vi "VISA_smu-buffer-new_with initialization.vi"(0 "VISA resource name in":refnum<visa-resource-name>, 3 "Voltage Source Level (V)":dbl, 7 "error in (no error)":errorcluster, 12 "End voltage":ext, 14 "Initial voltage":ext, 18 "Dark Current":bool) -> (20 "VISA resource name out":refnum<visa-resource-name>, 22 "F_I_Output (A)":dbl, 23 "S_I_Output (A)":string, 24 "F_V_Output (V)":dbl, 25 "S_V_Output (V)":string, 27 "error out":errorcluster)   [LabVIEW 2014]
panel:
  out "Numeric 2":i32
  out "Exp value":ext
  out "Exp value 2":ext
  out "floor(x): largest int <= x":ext
  out "Numeric":ext
  out "abs(x)":ext
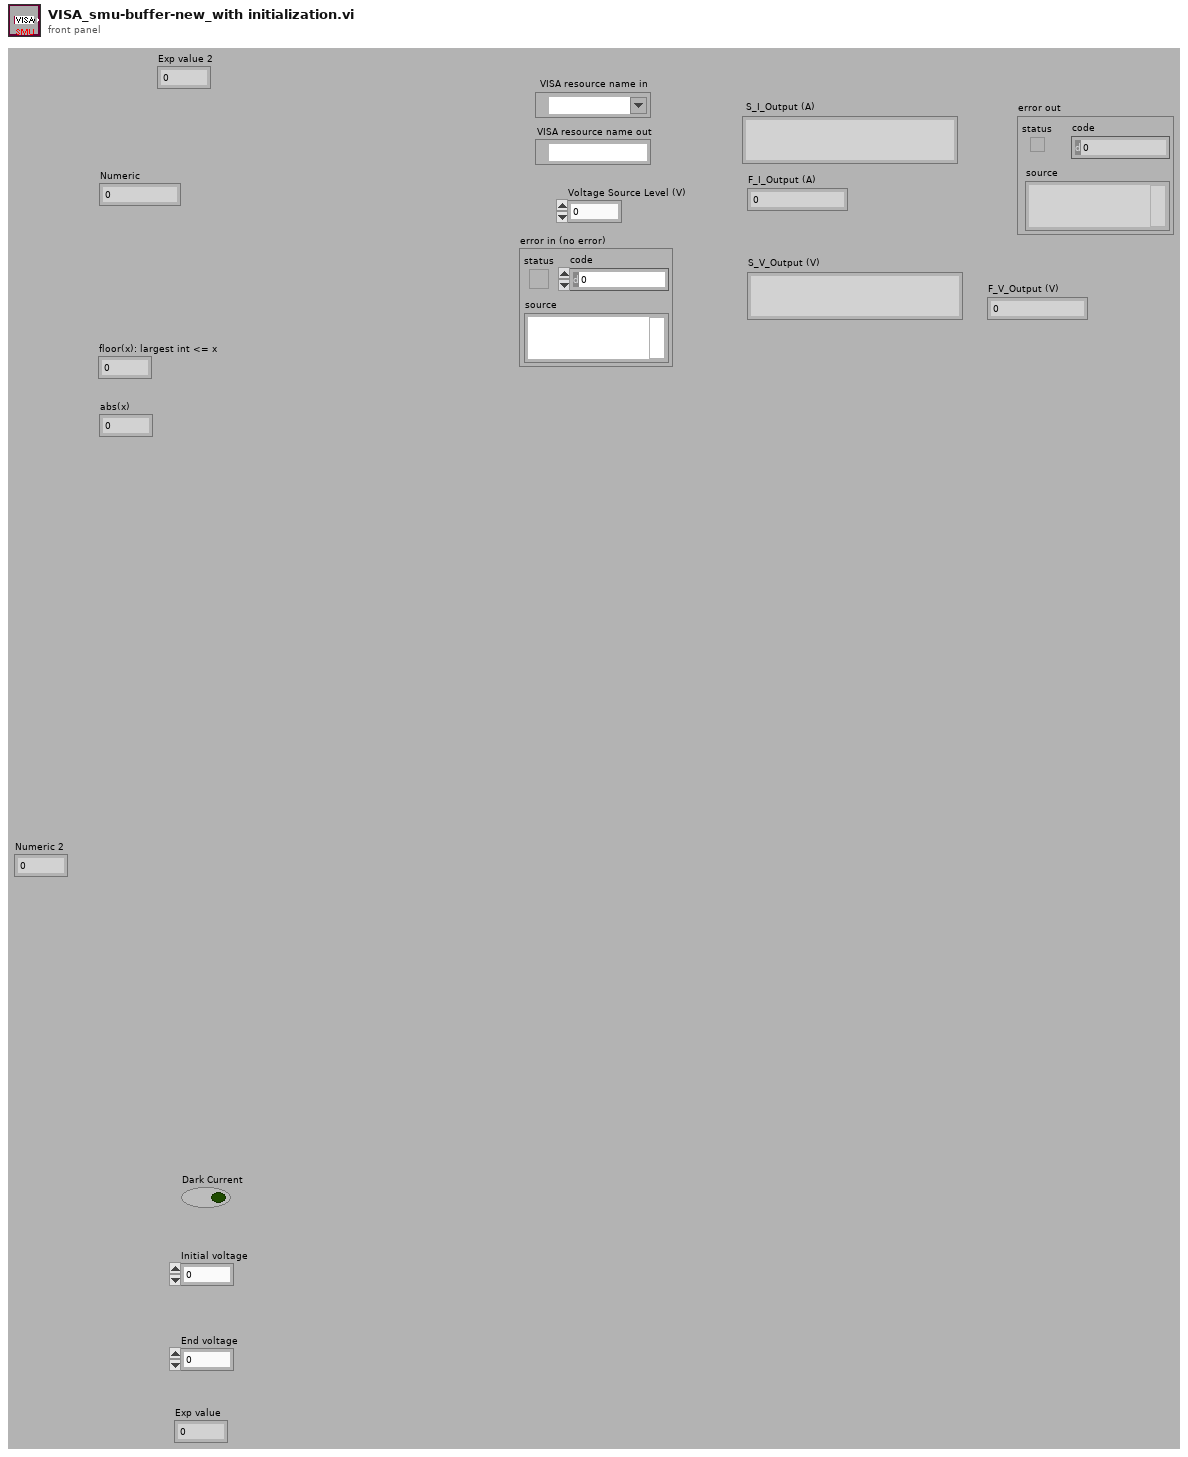
[diagram p1: front panel]
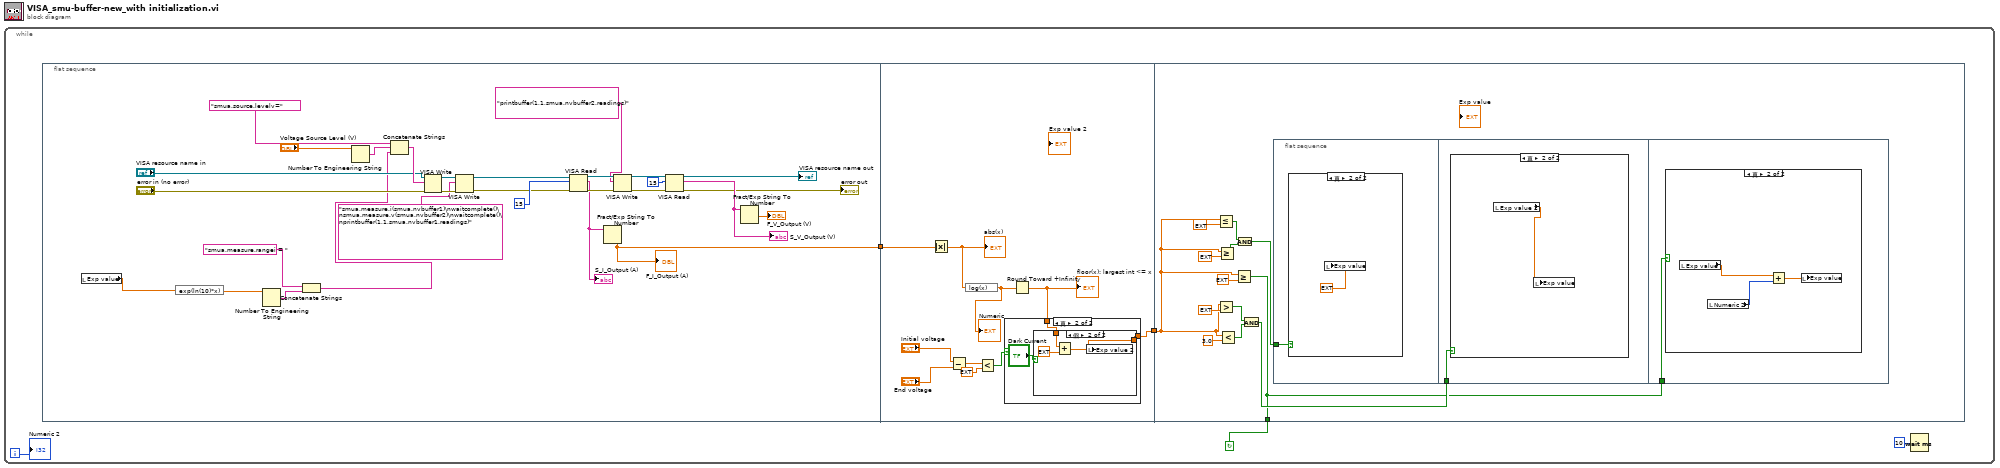
[diagram p0: block diagram]
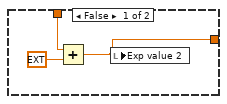
[diagram p2: hidden frame]
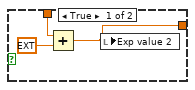
[diagram p3: hidden frame]
diagram:
  n1 = while {
    i -> [w3]
    stop <- w4 continue-if-true
    n2 = flat-sequence {
      tunnel: [w8] -> w1
      tunnel: [w40] -> w5
      tunnel: w1 -> [w41]
      tunnel: w5 -> [w58]
      tunnel: [w57] -> w4
      frame #0 {
        n3 = local read "Exp value"() -> (w6:ext)
        n4 = expression code="exp(ln(10)*x)"(w6) -> (w7:ext)
        n5 = Number To Engineering String(4:w7) -> (0:w17:string)  [unwired: 3 out]
        n6 = Concatenate Strings("smua.measure.rangei = " ("string"), w17) -> (w15:string)
        n7 = Number To Engineering String(4:"Voltage Source Level (V)") -> (0:w33:string)  [unwired: 3 out]
        n8 = Concatenate Strings("smua.source.levelv=", w33, w15) -> (w22:string)
        n9 = VISA Write(VISA resource name="VISA resource name in", write buffer=w22, error in (no error)="error in (no error)") -> (VISA resource name out=w24:refnum<visa-resource-name>, error out=w23:errorcluster)  [unwired: 1 out]
        n10 = VISA Write(VISA resource name=w24, write buffer="smua.measure.i(smua.nvbuffer1)\nwaitcomplete()\nsmua.measure.v(smua.nvbuffer2)\nwaitcomplete()\nprintbuffer(1,1,smua.nvbuffer1.readings)", error in (no error)=w23) -> (VISA resource name out=w14:refnum<visa-resource-name>, error out=w13:errorcluster)  [unwired: 1 out]
        n11 = VISA Read(VISA resource name=w14, byte count=u32 15, error in (no error)=w13) -> (VISA resource name out=w26:refnum<visa-resource-name>, read buffer=w25:string, error out=w27:errorcluster)  [unwired: 1 out]
        "S_I_Output (A)" <- w25
        n12 = Fract/Exp String To Number(string=w25) -> (number=w8:dbl)  [unwired: 4 out]
        "F_I_Output (A)" <- w8
        n13 = VISA Write(VISA resource name=w26, write buffer="printbuffer(1,1,smua.nvbuffer2.readings)", error in (no error)=w27) -> (VISA resource name out=w12:refnum<visa-resource-name>, error out=w11:errorcluster)  [unwired: 1 out]
        n14 = VISA Read(VISA resource name=w12, byte count=u32 15, error in (no error)=w11) -> (VISA resource name out=→"VISA resource name out":refnum<visa-resource-name>, read buffer=w29:string, error out=→"error out":errorcluster)  [unwired: 1 out]
        "S_V_Output (V)" <- w29
        n15 = Fract/Exp String To Number(string=w29) -> (number=→"F_V_Output (V)":dbl)  [unwired: 4 out]
      }
      frame #1 {
        n16 = Absolute Value(x=w41) -> (abs(x)=w43:dbl)
        "abs(x)" <- w43
        n17 = Subtract(x="Initial voltage", y="End voltage") -> (x-y=w37:ext)
        n18 = expression code="log(x)"(w43) -> (w44:dbl)
        "Numeric" <- w44
        n19 = Less?(x=w37, y=ext 0.0) -> (x < y?=w35:bool)
        n20 = Round Toward +Infinity(x=w44) -> (ceil(x): smallest int >= x=w42:dbl)
        "floor(x): largest int <= x" <- w42
        n21 = case shown="真" w35 {
          tunnel: w42 -> [w46 w50]
          tunnel: [w45 w49] -> w40
          frame False {
            n22 = Add(x=w46, y=ext 0.0) -> (x+y=w45:ext)
            n23 = local write "Exp value 2"(w45) -> ()
          }
          frame True {
            n24 = case shown="假" "Dark Current" {
              tunnel: w50 -> [w52 w55]
              tunnel: [w51 w54] -> w49
              frame True {
                n25 = Add(x=w52, y=ext 0.0) -> (x+y=w51:ext)
                n26 = local write "Exp value 2"(w51) -> ()
              }
              frame False {
                n27 = Add(x=w55, y=ext 1.0) -> (x+y=w54:ext)
                n28 = local write "Exp value 2"(w54) -> ()
              }
            }
          }
        }
      }
      frame #2 {
        n29 = Less Or Equal?(x=w58, y=ext -14.0) -> (x <= y?=w62:bool)
        n30 = Greater?(x=w58, y=ext -12.0) -> (0:w67:bool)
        n31 = Greater Or Equal?(x=w58, y=ext -20.0) -> (x >= y?=w61:bool)
        n32 = Less?(x=w58, y=3.0) -> (x < y?=w66:bool)
        n33 = Greater Or Equal?(x=w58, y=ext 3.0) -> (x >= y?=w57:bool)
        n34 = And(x=w62, y=w61) -> (x .and. y?=w63:bool)
        n35 = And(x=w67, y=w66) -> (x .and. y?=w68:bool)
        n36 = flat-sequence {
          tunnel: w63 -> [w70]
          tunnel: w68 -> [w72]
          tunnel: w57 -> [w74]
          frame #0 {
            n37 = case shown="真" w70 {
              frame False {
              }
              frame True {
                n38 = local write "Exp value"(ext -14.0 ("Exp value")) -> ()
              }
            }
          }
          frame #1 {
            n39 = case shown="真" w72 {
              frame False {
              }
              frame True {
                n40 = local read "Exp value 2"() -> (w73:ext)
                n41 = local write "Exp value"(w73) -> ()
              }
            }
          }
          frame #2 {
            n42 = case shown="真" w74 {
              frame False {
              }
              frame True {
                n43 = local read "Exp value"() -> (w75:ext)
                n44 = local read "Numeric 2"() -> (w77:i32)
                n45 = Add(x=w75, y=w77) -> (x+y=w76:ext)
                n46 = local write "Exp value"(w76) -> ()
              }
            }
          }
        }
      }
    }
    n47 = Wait (ms)(milliseconds to wait=u32 10) -> ()  [unwired: 1 out]
    "Numeric 2" <- w3
  }
